vi "Test_Fault_Reset.vi"() -> ()   [LabVIEW 2016, in "Motor Base.lvlib"]
uses:
  Motor Base.lvlib
panel:
  out "Transmit PDO mapping 1-Error code":u16
  out "Transmit PDO mapping 1-Statusword":u16 format="%b"
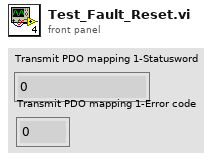
[diagram p1: front panel]
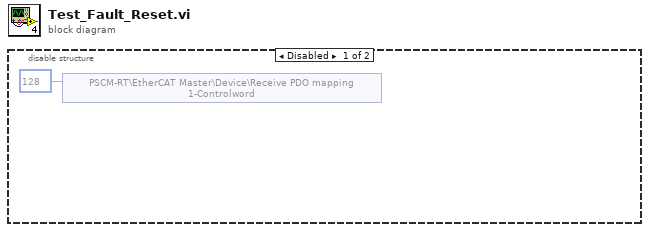
[diagram p0: block diagram]
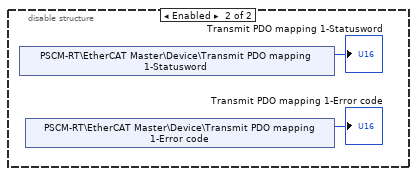
[diagram p2: hidden frame]
diagram:
  n1 = disable-structure shown="Disabled" {
    frame Disabled {
      n2 = shared-variable "PSCM-RT\\EtherCAT Master\\Device\\Receive PDO mapping 1-Controlword"(u16 128 ("Receive PDO mapping 1-Controlword")) -> ()  [unwired: 1 in, 1 out]
    }
    frame Enabled {
      n3 = shared-variable "PSCM-RT\\EtherCAT Master\\Device\\Transmit PDO mapping 1-Statusword"() -> (→"Transmit PDO mapping 1-Statusword":u16)  [unwired: 1 in, 1 out]
      n4 = shared-variable "PSCM-RT\\EtherCAT Master\\Device\\Transmit PDO mapping 1-Error code"() -> (→"Transmit PDO mapping 1-Error code":u16)  [unwired: 1 in, 1 out]
    }
  }
